vi "Creat DataColumn by Name and Type.vi"(8 "error in (no error)":errorcluster caption="错误输入（无错误）", 9 "anything":variant, 10 "columnName":string, 11 "Data Column 输入":refnum<class "Data Column.lvclass"> caption="DNL_LabVIEW Object in") -> (0 "error out":errorcluster caption="错误输出", 3 "Data Column 输出":refnum<class "Data Column.lvclass"> caption="DNL_LabVIEW Object out")   [LabVIEW 2012, in "Data Grid VIEW.lvlib" / "Data Column.lvclass"]
uses:
  Data Column.lvclass
  System.Data
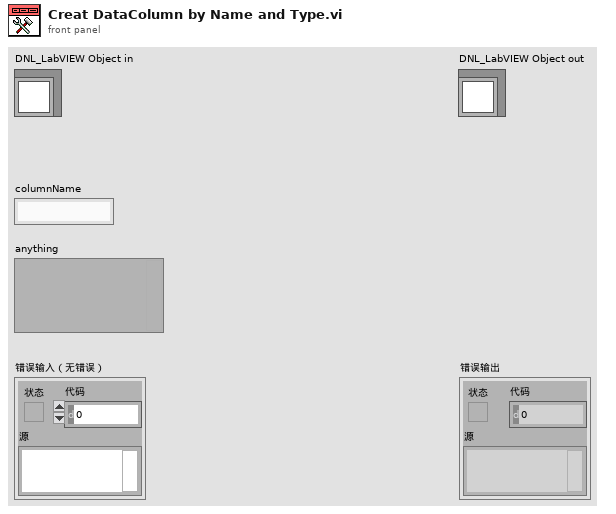
[diagram p1: front panel]
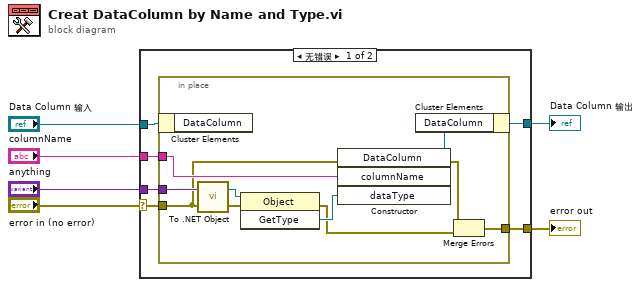
[diagram p0: block diagram]
diagram:
  n1 = case shown="无错误" "error in (no error)" {
    selector: "error in (no error)" -> [w10 w24]
    tunnel: [w9 w24] -> w5
    tunnel: [w11 w23] -> w3
    tunnel: "Data Column 输入" -> [w12 w23]
    tunnel: "columnName" -> [w8 _]
    tunnel: "anything" -> [w7 _]
    frame No Error {
      n2 = in-place {
        in-place-border: w10 -> [w16]
        in-place-border: [w13] -> w9
        in-place-border: w8 -> [w21]
        in-place-border: w7 -> [w17]
        n3 = in-place-cluster #1(w12) -> ()  [unwired: 1 out]
        n4 = call <vilib>:"To .NET Object.vi"("error in (no error)"=w16, "anything"=w17) -> ("error out"=w19:errorcluster, ".NET object"=w18:refnum<k24>)
        n5 = invoke class="Object" method="GetType"(reference=w18, error in=w19) -> (error out=w14:errorcluster, "GetType"=w20:refnum<k24>)  [unwired: 1 in, 1 out]
        n6 = constructor class="DataColumn"(error in=w16, "columnName"=w21, "dataType"=w20) -> (reference out=w22:refnum<k24>, error out=w15:errorcluster)  [unwired: 2 in, 3 out]
        n7 = in-place-cluster #1("DataColumn"=w22) -> (w11:refnum<class "Data Column.lvclass">)
        n8 = Merge Errors(w15, w14) -> (w13:errorcluster)
      }
    }
    frame Error {
    }
  }
  "error out" <- w5
  "Data Column 输出" <- w3
